vi "Set Home Search Mode.vi"(4 "Home mode":T1(ring)=enum."Find Home Signal", 5 "error in (no error)":errorcluster, 7 "Axis (1)":i32=1 min=1 max=3, 8 "VISA resource name":refnum<visa-resource-name>) -> (0 "error out":errorcluster, 3 "VISA resource name out":refnum<visa-resource-name>)   [LabVIEW 2019, in "Newport ESP301.lvlib"]
doc: "This command selects the home search type without invoking the home search sequence (see the description of OR command for more information on home search). The seven home search types are +0 Position Count, Home Switch and Index Signals, Home Switch Signal, Positive Limit Signal, Negative Limit Signal, Positive Limit and Index Signals and Negative Limit and Index Signals.\n\nThe \"home search mode\" parameter is overwritten by the \"Search For Home.vi\" command parameter."
uses:
  Newport ESP301.lvlib
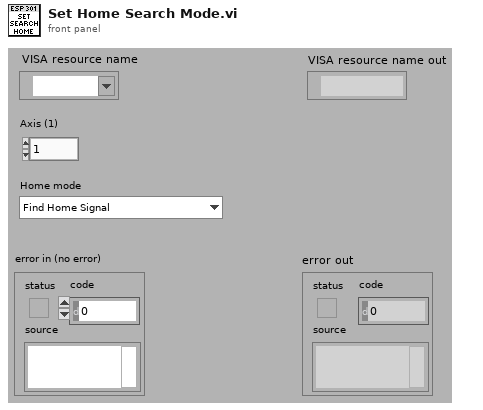
[diagram p1: front panel]
types:
  T1 = enum16{"Find +0 Position Count", "Find Home and Index Signals", "Find Home Signal", "Find Positive Limit Signal", "Find Negative Limit Signal", "Find Positve Limit and Index Signals", "Find Negative Limit and Index Signals"}
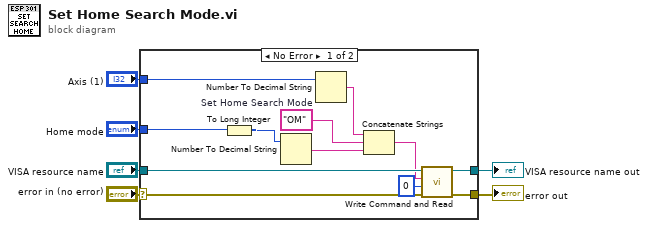
[diagram p0: block diagram]
diagram:
  n1 = case shown="No Error" "error in (no error)" {
    selector: "error in (no error)" -> [w17 w20]
    tunnel: [w16 w20] -> w5
    tunnel: "VISA resource name" -> [w18 w19]
    tunnel: [w15 w19] -> w3
    tunnel: "Axis (1)" -> [w11 _]
    tunnel: "Home mode" -> [w8 _]
    frame No Error {
      w13 = "OM"  # Set Home Search Mode
      n2 = To Long Integer(number=w8) -> (32bit integer=w7:i32)
      n3 = Number To Decimal String(number=w7) -> (decimal integer string=w14:string)  [unwired: 1 in]
      n4 = Number To Decimal String(number=w11) -> (decimal integer string=w12:string)  [unwired: 1 in]
      n5 = Concatenate Strings(w12, w13, w14) -> (w10:string)
      n6 = call "Write Command and Read.vi"("error in (no error)"=w17, "Bytes to read (100)"=u32 0, "Command"=w10, "VISA resource name"=w18) -> ("error out"=w16:errorcluster, "VISA resource name out"=w15:refnum<visa-resource-name>)  [unwired: 3 in, 1 out]
    }
    frame Error {
    }
  }
  "error out" <- w5
  "VISA resource name out" <- w3
